vi "StateDrivebase.vi"(0 "Master State":enum16{"Normal", "Climb"}(ring)) -> ()   [LabVIEW 2020]
doc: "This VI performs all of the calculations and decisions related to the swerve drive. Driver profiles are tuned from this front panel."
uses:
  <vilib>/Rock Robotics/WPI/DriverStation/WPI_DriverStationRobotMode2.ctl
  drivercommands.vi
  driverdata.vi
  sensordata.vi
  robotoutputs.vi
  robotconstants.vi
  autonomousinfo.vi
panel:
  in  "Max Strafing While Climbing":dbl=0.25
  in  "Shooting Decceleration Limit (/s)":dbl=2.25
  in  "Slew Rate Limit (/s)":dbl=2.25
  in  "Max Strafing While Shooting":dbl=0.25
  in  "PID Tuning Anti-Drift":T1={"Kp"=0.00045, "Ki"=0.0, "Kd"=0.0, "N-Diff"=3, "N-Int"=10, "Int Error Window"=90.0, "Max Ouput"=1.0, "Min Output"=-1.0, "Square Derivative"=FALSE, "N-Prop"=5} {"N-Prop" min=1; "Int Error Window" min=0.0; "N-Int" min=2; "N-Diff" min=2; "Kd" min=0.0; "Ki" min=0.0; "Kp" min=0.0}
  in  "Anti-Drift Deceleration Hysteresis (ms)":u32=1
  out "Anti-Drift Control":bool
  in  "Anti-Drift Strafe Deadband (ft/s)":dbl=3.0
  in  "Manually Disable Anti-Drift":bool
  in  "PID Tuning Heading Lock":T2={"Kp"=0.0045, "Ki"=0.01, "Kd"=0.0002, "N-Diff"=10, "N-Int"=10, "Int Error Window"=30.0, "Max Ouput"=1.0, "Min Output"=-1.0} {"Int Error Window" min=0.0; "N-Int" min=2; "N-Diff" min=2; "Kd" min=0.0; "Ki" min=0.0; "Kp" min=0.0}
  out "Heading Controller Summary":T3(graph)
  in  "Manual Fudge Factor Heading Lock (deg)":dbl=10.0
  in  "Plot Heading PID":bool
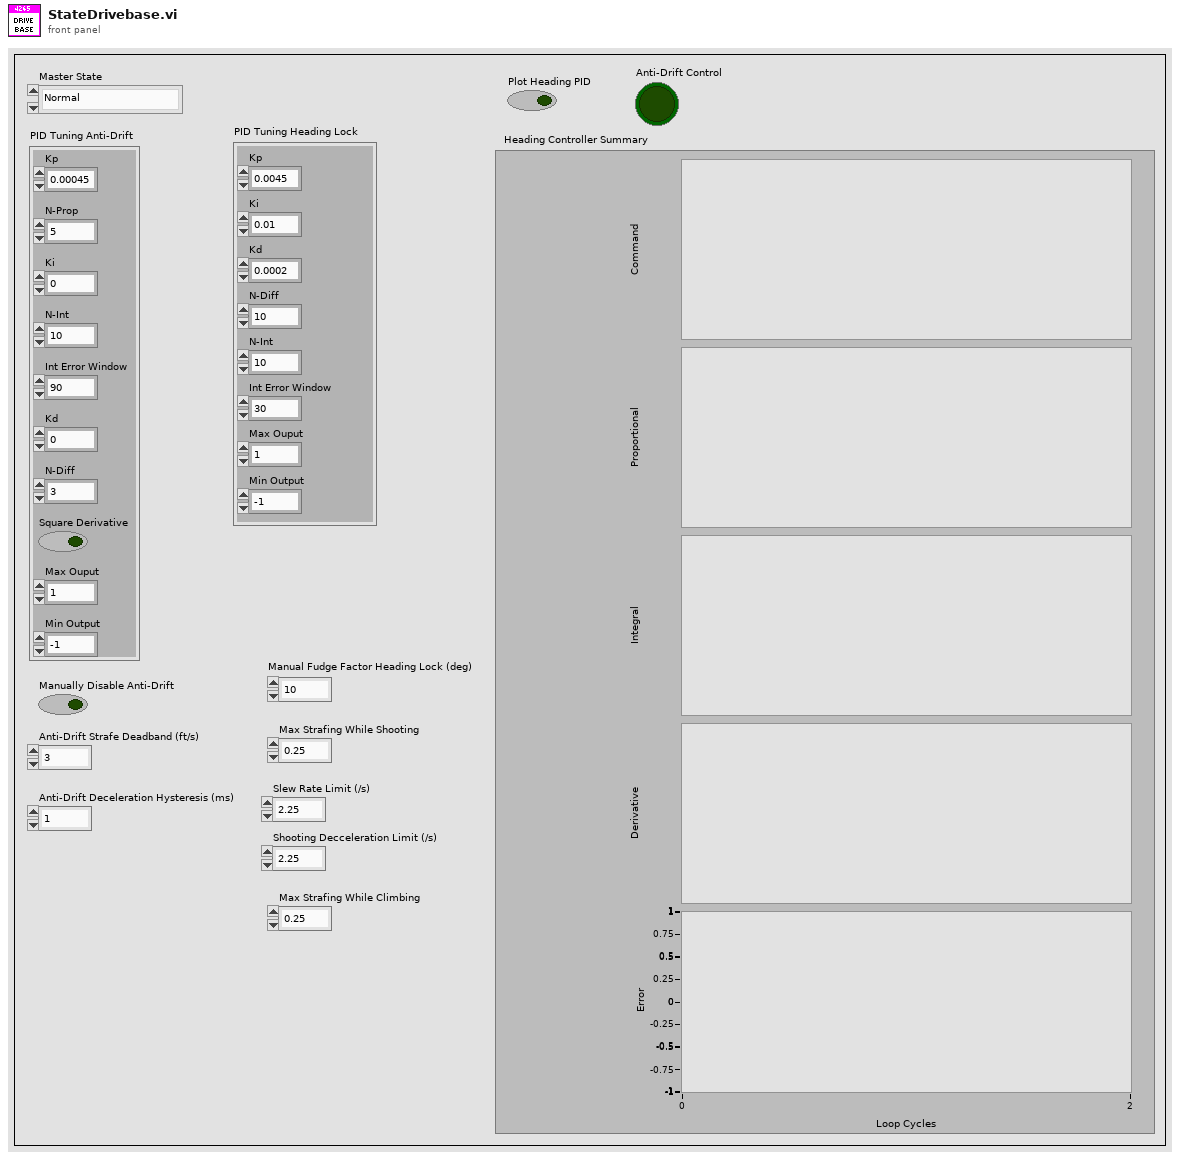
[diagram p1: front panel]
types:
  T1 = cluster{"Kp":dbl, "Ki":dbl, "Kd":dbl, "N-Diff":i32, "N-Int":i32, "Int Error Window":dbl, "Max Ouput":dbl, "Min Output":dbl, "Square Derivative":bool, "N-Prop":i32}
  T2 = cluster{"Kp":dbl, "Ki":dbl, "Kd":dbl, "N-Diff":i32, "N-Int":i32, "Int Error Window":dbl, "Max Ouput":dbl, "Min Output":dbl}
  T3 = cluster{"Command":dbl, "Proportional":dbl, "Integral":dbl, "Derivative":dbl, "Goal":dbl}
  T4 = typedef "WPI_DriverStationRobotMode2.ctl" = enum16{"Autonomous Disabled", "Autonomous Enabled", "Teleop Disabled", "Teleop Enabled", "Disconnected", "Finish", "Test Disabled", "Test Enabled", "Emergency Stopped"}
  T5 = cluster{"Current Setpoints[0]":dbl, "Current Setpoints[1]":dbl, "Current Setpoints[2]":dbl, "Current Setpoints[3]":dbl, "Current Setpoints[4]":dbl, "Current Setpoints[5]":dbl, "Current Setpoints[6]":dbl, "Current Setpoints[7]":dbl, "Current Setpoints[8]":dbl}
  T6 = enum16{"Robot-Oriented", "Field-Oriented", "Intake"}
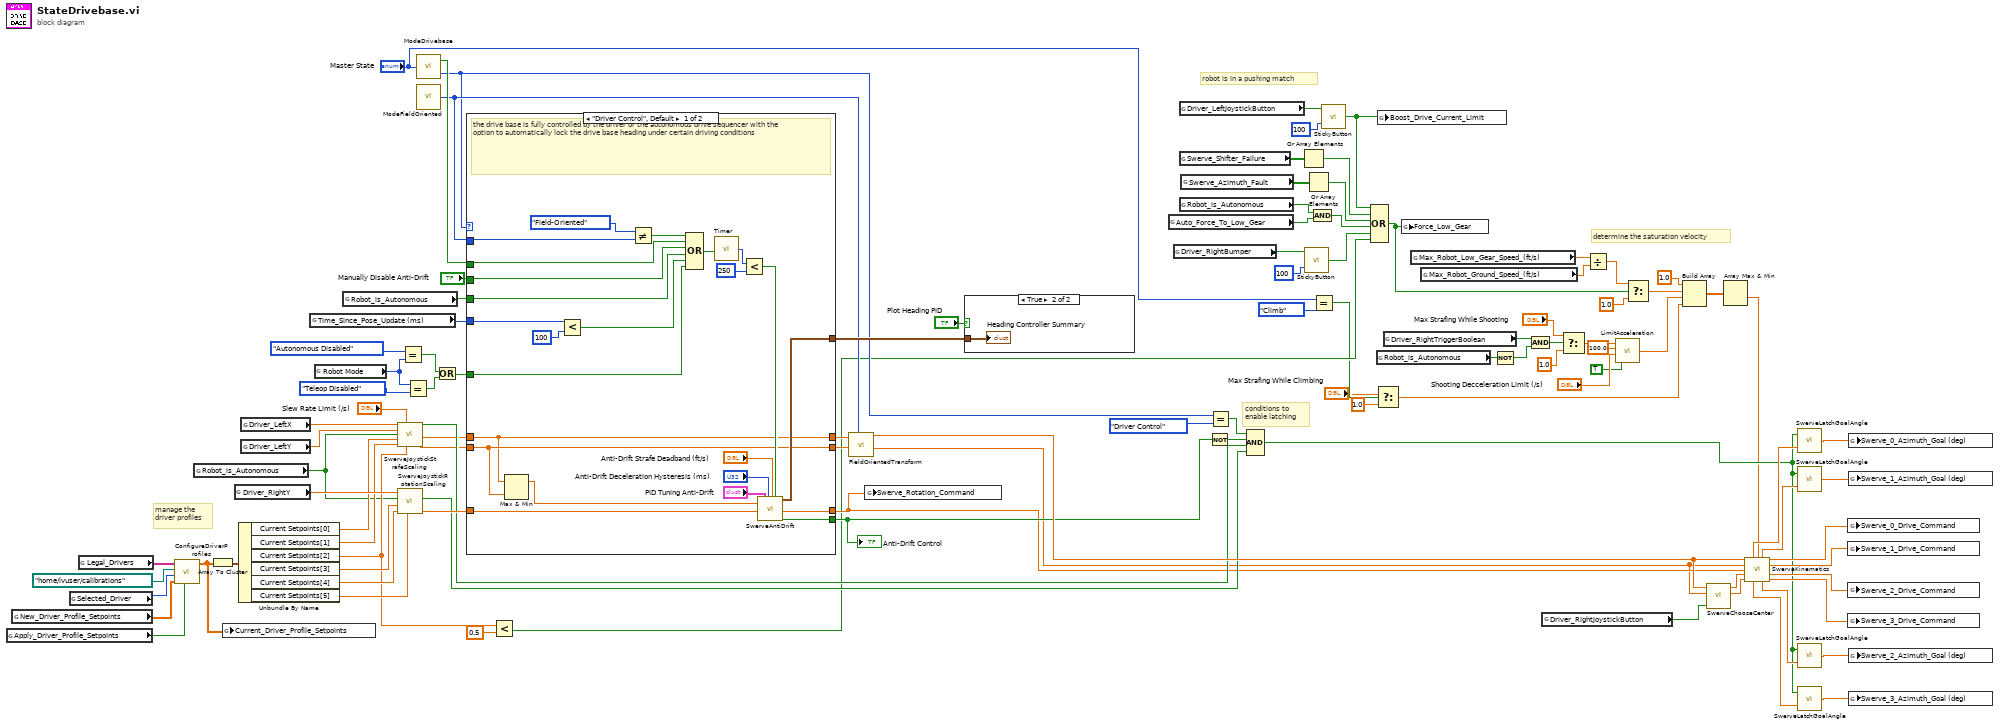
[diagram p0: block diagram]
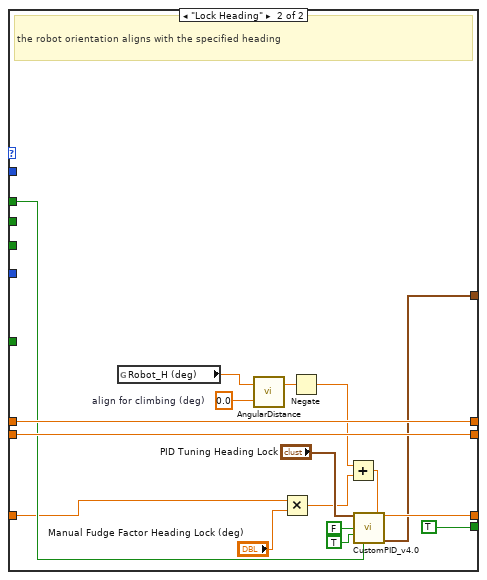
[diagram p3: hidden frame]
diagram:
  # "determine the saturation velocity"
  # "robot is in a pushing match"
  # "conditions to\nenable latching"
  # "manage the\ndriver profiles"
  n1 = global read "driverdata.vi" "Apply_Driver_Profile_Setpoints"() -> (w51:bool)
  n2 = global read "driverdata.vi" "New_Driver_Profile_Setpoints"() -> (w53:dbl[])
  n3 = global read "driverdata.vi" "Selected_Driver"() -> (w52:i32)
  n4 = global read "robotconstants.vi" "Legal_Drivers"() -> (w46:string[])
  n5 = call "ConfigureDriverProfiles.vi"("Apply New Setpoint"=w51, "New Setpoints"=w53, "Selected Driver"=w52, "Setpoint Save Location"=path "/home/lvuser/calibrations", "Driver Profile Names"=w46) -> ("Current Setpoints"=w50:dbl[])  [unwired: 6 in]
  n6 = global read "driverdata.vi" "Robot_is_Autonomous"() -> (w42:bool)
  n7 = Array To Cluster(array=w50) -> (cluster=w49:T5)
  n8 = global write "robotoutputs.vi" "Current_Driver_Profile_Setpoints"(w50) -> ()
  n9 = global read "drivercommands.vi" "Driver_RightY"() -> (w86:dbl)
  n10 = Unbundle By Name(w49) -> ("Current Setpoints[0]"=w75:dbl, "Current Setpoints[1]"=w74:dbl, "Current Setpoints[2]"=w45:dbl, "Current Setpoints[3]"=w63:dbl, "Current Setpoints[4]"=w62:dbl, "Current Setpoints[5]"=w61:dbl)
  n11 = global read "drivercommands.vi" "Driver_LeftX"() -> (w89:dbl)
  n12 = global read "drivercommands.vi" "Driver_LeftY"() -> (w88:dbl)
  n13 = global read "sensordata.vi" "Time_Since_Pose_Update (ms)"() -> (w97:u32)
  n14 = global read "driverdata.vi" "Robot Mode"() -> (w68:T4)
  n15 = global read "driverdata.vi" "Robot_is_Autonomous"() -> (w96:bool)
  n16 = call "SwerveJoystickStrafeScaling.vi"("Raw Joystick X"=w89, "Slew Rate Limit (/s)"="Slew Rate Limit (/s)", "Raw Joystick Y"=w88, "Auto Control"=w42, "Strafe Deadband"=w75, "Strafe Scaling"=w74, "Strafe Maximum"=w45) -> ("In Deadband"=w82:bool, "Scaled Joystick X"=w27:dbl, "Scaled Joystick Y"=w36:dbl)  [unwired: 6 in]
  n17 = call "SwerveJoystickRotationScaling.vi"("Rotation Maximum"=w61, "Rotation Scaling"=w62, "Rotation Deadband"=w63, "Auto Control"=w42, "Raw Joystick Rotation"=w86) -> ("Scaled Joystick Rotation"=w87:dbl, "In Deadband"=w83:bool)  [unwired: 4 in]
  n18 = Equal?(x=WPI_DriverStationRobotMode2."Autonomous Disabled" ("Robot Mode"), y=w68) -> (x = y?=w66:bool)
  n19 = Equal?(x=w68, y=WPI_DriverStationRobotMode2."Teleop Disabled" ("Robot Mode")) -> (x = y?=w65:bool)
  n20 = call "ModeDrivebase.vi"("Master State"="Master State") -> ("Drive Mode Change"=w94:bool, "Drive Mode"=w57:enum16{"Driver Control", "Lock Heading"})
  n21 = call "ModeFieldOriented.vi"() -> ("Orientation Mode"=w77:T6)  [unwired: 1 in]
  n22 = Or(x=w66, y=w65) -> (x .or. y?=w64:bool)
  n23 = case shown="\"Driver Control\", Default" w57 {
    tunnel: [w107 w142] -> w76
    tunnel: [w106 w140] -> w103
    tunnel: w27 -> [w106 w140]
    tunnel: w36 -> [w107 w142]
    tunnel: w87 -> [w118 w132]
    tunnel: [w119 w139] -> w81
    tunnel: [w124 TRUE ("auto rot control")] -> w84
    tunnel: w77 -> [w125 _]
    tunnel: w96 -> [w122 _]
    tunnel: w94 -> [w116 w135]
    tunnel: w97 -> [w127 _]
    tunnel: [w121 w134] -> w95
    tunnel: "Manually Disable Anti-Drift" -> [w120 _]
    tunnel: w64 -> [w110 _]
    frame "Driver Control", Default {
      # "the drive base is fully controlled by the driver or the autonomous drive sequencer with the option to automatically lock the drive base heading under certain driving conditions"
      n24 = Max & Min(x=w106, y=w107) -> (max(x,y)=w105:dbl)  [unwired: 1 out]
      n25 = Less?(x=w127, y=u32 100) -> (x < y?=w123:bool)
      n26 = Not Equal?(x=T6."Field-Oriented", y=w125) -> (x != y?=w115:bool)
      n27 = Compound Arithmetic op=OR(w115, w116, w120, w122, w123, w110) -> (w113:bool)
      n28 = call "Timer.vi"("Reset Timer"=w113) -> ("Time (ms)"=w114:u32)
      n29 = Less?(x=w114, y=u32 250) -> (x < y?=w111:bool)
      n30 = call "SwerveAntiDrift.vi"("Max Driver Translation Joystick"=w105, "Driver Rotation Joystick"=w118, "PID Tuning Parameters"="PID Tuning Anti-Drift", "Deceleration Hysteresis (ms)"="Anti-Drift Deceleration Hysteresis (ms)", "Strafe Deadband (ft/s)"="Anti-Drift Strafe Deadband (ft/s)", "External Disables"=w111) -> ("Controller Summary"=w121:T3, "Joystick Rotation"=w119:dbl, "Anti-Drift"=w124:bool)  [unwired: 11 in]
    }
    frame "Lock Heading" {
      w143 = 0.0  # align for climbing (deg)
      # "the robot orientation aligns with the specified heading"
      n31 = global read "sensordata.vi" "Robot_H (deg)"() -> (w144:dbl)
      n32 = call "AngularDistance.vi"("Goal Angle (deg) [0,360]"=w143, "Current Angle (deg) [-Inf,+Inf]"=w144) -> ("Signed Angular Distance (deg) [-180,+180]"=w133:dbl)  [unwired: 1 out]
      n33 = Multiply(x=w132, y="Manual Fudge Factor Heading Lock (deg)") -> (x*y=w131:dbl)
      n34 = Negate(x=w133) -> (-x=w130:dbl)
      n35 = Add(x=w130, y=w131) -> (x+y=w129:dbl)
      n36 = call "CustomPID_v4.0.vi"("PID Tuning Parameters"="PID Tuning Heading Lock", "Custom Error Calculation"=w129, "Reset on Goal Change ?"=FALSE, "Use Custom Error Calculation ?"=TRUE, "Reinit"=w135) -> ("Command"=w139:dbl, "Controller Summary"=w134:T3)  [unwired: 7 in, 2 out]
    }
  }
  "Anti-Drift Control" <- w84
  n37 = Less?(x=w45, y=0.5) -> (x < y?=w7:bool)
  n38 = call "FieldOrientedTransform.vi"("Orientation Mode"=w77, "Joystick Y"=w76, "Joystick X"=w103) -> ("Joystick Y'"=w78:dbl, "Joystick X'"=w85:dbl)  [unwired: 7 in]
  n39 = global write "robotoutputs.vi" "Swerve_Rotation_Command"(w81) -> ()
  n40 = case shown="True" "Plot Heading PID" {
    tunnel: w95 -> [_ w145]
    frame False {
    }
    frame True {
      "Heading Controller Summary" <- w145
    }
  }
  n41 = global read "autonomousinfo.vi" "Auto_Force_To_Low_Gear"() -> (w24:bool)
  n42 = global read "drivercommands.vi" "Driver_RightBumper"() -> (w60:bool)
  n43 = global read "drivercommands.vi" "Driver_LeftJoystickButton"() -> (w91:bool)
  n44 = global read "sensordata.vi" "Swerve_Shifter_Failure"() -> (w26:bool[])
  n45 = global read "driverdata.vi" "Robot_is_Autonomous"() -> (w23:bool)
  n46 = global read "sensordata.vi" "Swerve_Azimuth_Fault"() -> (w25:bool[])
  n47 = Not(x=w84) -> (.not. x?=w80:bool)
  n48 = Equal?(x=w57, y=enum16{"Driver Control", "Lock Heading"}."Driver Control" ("Drive Mode")) -> (x = y?=w79:bool)
  n49 = Compound Arithmetic op=AND(w79, w80, w82, w83) -> (w14:bool)
  n50 = Or Array Elements(Boolean array=w26) -> (logical OR=w20:bool)
  n51 = call "StickyButton.vi"("Time threshold (ms)"=u32 100 ("y"), "Button Input"=w60) -> ("Sticky Button"=w58:bool)
  n52 = Or Array Elements(Boolean array=w25) -> (logical OR=w21:bool)
  n53 = And(x=w23, y=w24) -> (x .and. y?=w22:bool)
  n54 = Equal?(x="Master State", y=enum16{"Normal", "Climb"}."Climb") -> (x = y?=w6:bool)
  n55 = call "StickyButton.vi"("Time threshold (ms)"=u32 100 ("y"), "Button Input"=w91) -> ("Sticky Button"=w19:bool)
  n56 = Compound Arithmetic op=OR(w19, w20, w21, w22, w58, w7) -> (w34:bool)
  n57 = global read "driverdata.vi" "Robot_is_Autonomous"() -> (w35:bool)
  n58 = Select(t="Max Strafing While Climbing", s=w6, f=1.0) -> (s? t:f=w1:dbl)
  n59 = global write "robotoutputs.vi" "Boost_Drive_Current_Limit"(w19) -> ()
  n60 = global read "drivercommands.vi" "Driver_RightTriggerBoolean"() -> (w44:bool)
  n61 = global write "robotoutputs.vi" "Force_Low_Gear"(w34) -> ()
  n62 = global read "robotconstants.vi" "Max_Robot_Low_Gear_Speed_(ft/s)"() -> (w30:dbl)
  n63 = global read "robotconstants.vi" "Max_Robot_Ground_Speed_(ft/s)"() -> (w29:dbl)
  n64 = Not(x=w35) -> (.not. x?=w43:bool)
  n65 = And(x=w44, y=w43) -> (x .and. y?=w32:bool)
  n66 = global read "drivercommands.vi" "Driver_RightJoystickButton"() -> (w93:bool)
  n67 = Select(t="Max Strafing While Shooting", s=w32, f=1.0) -> (s? t:f=w12:dbl)
  n68 = Divide(x=w30, y=w29) -> (x/y=w28:dbl)
  n69 = call "LimitAcceleration.vi"("Apply Limit"=TRUE, "Decceleration Limit (/s)"="Shooting Decceleration Limit (/s)", "Acceleration Limit (/s)"=100.0, "Raw Input"=w12) -> ("Output"=w11:dbl)
  n70 = Select(t=w28, s=w34, f=1.0) -> (s? t:f=w17:dbl)
  n71 = Build Array(1.0 ("element"), w17, w11, w1) -> (w18:dbl[])
  n72 = call "SwerveChooseCenter.vi"("Defensive Driving Trigger"=w93, "Joystick Y"=w78, "Joystick X"=w85) -> ("Cy (in)"=w55:dbl, "Cx (in)"=w56:dbl)  [unwired: 5 in]
  n73 = Array Max & Min(array=w18) -> (min value=w13:dbl)  [unwired: 3 out]
  n74 = call "SwerveKinematics.vi"("Joystick X"=w85, "Saturation Velocity (ul)"=w13, "Joystick Y"=w78, "Joystick Rotation"=w81, "Cx (in)"=w56, "Cy (in)"=w55) -> ("Module 0 Angle (deg)"=w102:dbl, "Module 1 Angle (deg)"=w101:dbl, "Module 0 Velocity Command (ul)"=w73:dbl, "Module 1 Velocity Command (ul)"=w72:dbl, "Module 2 Velocity Command (ul)"=w71:dbl, "Module 3 Angle (deg)"=w98:dbl, "Module 2 Angle (deg)"=w99:dbl, "Module 3 Velocity Command (ul)"=w70:dbl)  [unwired: 2 in]
  n75 = call "SwerveLatchGoalAngle.vi"("Raw Goal Angle"=w102, "In Deadband"=w14) -> ("Latched Goal Angle"=w41:dbl)
  n76 = call "SwerveLatchGoalAngle.vi"("Raw Goal Angle"=w101, "In Deadband"=w14) -> ("Latched Goal Angle"=w40:dbl)
  n77 = call "SwerveLatchGoalAngle.vi"("Raw Goal Angle"=w99, "In Deadband"=w14) -> ("Latched Goal Angle"=w39:dbl)
  n78 = call "SwerveLatchGoalAngle.vi"("Raw Goal Angle"=w98, "In Deadband"=w14) -> ("Latched Goal Angle"=w38:dbl)
  n79 = global write "robotoutputs.vi" "Swerve_0_Drive_Command"(w73) -> ()
  n80 = global write "robotoutputs.vi" "Swerve_1_Drive_Command"(w72) -> ()
  n81 = global write "robotoutputs.vi" "Swerve_2_Drive_Command"(w71) -> ()
  n82 = global write "robotoutputs.vi" "Swerve_3_Drive_Command"(w70) -> ()
  n83 = global write "robotoutputs.vi" "Swerve_0_Azimuth_Goal (deg)"(w41) -> ()
  n84 = global write "robotoutputs.vi" "Swerve_1_Azimuth_Goal (deg)"(w40) -> ()
  n85 = global write "robotoutputs.vi" "Swerve_2_Azimuth_Goal (deg)"(w39) -> ()
  n86 = global write "robotoutputs.vi" "Swerve_3_Azimuth_Goal (deg)"(w38) -> ()
